vi "CollectorWrap.vi"(7 "Action":T1=enum."Collect", 8 "error in":errorcluster) -> (0 "error out":errorcluster)   [LabVIEW 2013]
uses:
  CollectorWrapAction.ctl
  DoubleSolenoidAction.ctl
  RollerAction.ctl
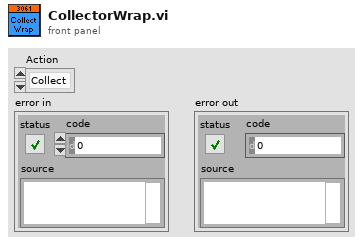
[diagram p1: front panel]
types:
  T1 = typedef "CollectorWrapAction.ctl" = enum16{"PreCollect", "Collect", "Stop"}
  T2 = typedef "DoubleSolenoidAction.ctl" = enum16{"Init", "Middle", "In", "Out"}
  T3 = typedef "RollerAction.ctl" = enum16{"Init", "Off", "Forward", "Reverse"}
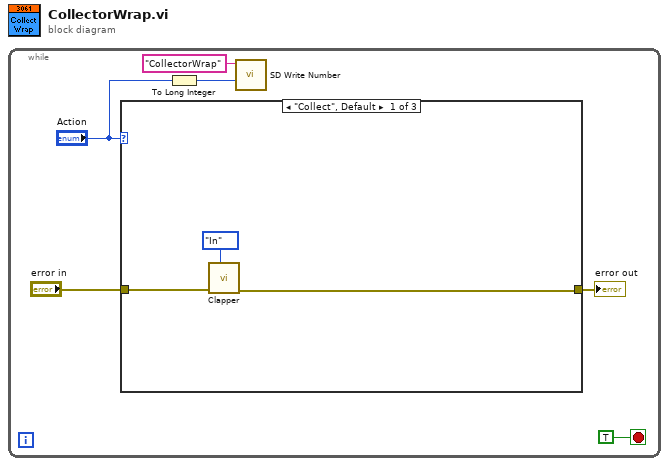
[diagram p0: block diagram]
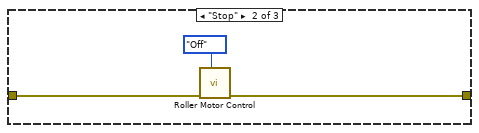
[diagram p2: hidden frame]
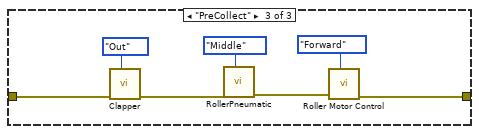
[diagram p3: hidden frame]
diagram:
  n1 = while {
    stop <- TRUE stop-if-true
    n2 = case shown="\"Collect\", Default" "Action" {
      tunnel: "error in" -> [w9 w12 w17]
      tunnel: [w8 w11 w19] -> w4
      frame "Collect", Default {
        n3 = call "Clapper.vi"("State"=DoubleSolenoidAction."In", "Error in"=w9) -> ("Error out"=w8:errorcluster)  [unwired: 9 in]
      }
      frame "Stop" {
        n4 = call "Roller Motor Control.vi"("Action"=RollerAction."Off", "Error in"=w12) -> ("Error out"=w11:errorcluster)  [unwired: 9 in]
      }
      frame "PreCollect" {
        n5 = call "Clapper.vi"("State"=DoubleSolenoidAction."Out", "Error in"=w17) -> ("Error out"=w16:errorcluster)  [unwired: 9 in]
        n6 = call "RollerPneumatic.vi"("State"=DoubleSolenoidAction."Middle", "Error in"=w16) -> ("Error out"=w15:errorcluster)  [unwired: 9 in]
        n7 = call "Roller Motor Control.vi"("Action"=RollerAction."Forward", "Error in"=w15) -> ("Error out"=w19:errorcluster)  [unwired: 9 in]
      }
    }
    "error out" <- w4
    n8 = To Long Integer(number="Action") -> (32bit integer=w3:i32)
    n9 = call <vilib>:"SD Write Number.vi"("Numeric"=w3, "Name"="CollectorWrap") -> ()  [unwired: 8 in, 2 out]
  }
